vi "HEWH Decision Logic Cutout Cutin.vi"(6 "Cut Out Timer (Over)":bool, 8 "Error In":errorcluster, 9 "Bottom":bool, 10 "Cut In Timer (Over)":bool, 11 "Top":bool) -> (0 "Error Out":errorcluster, 3 "Output":bool)   [LabVIEW 2023]
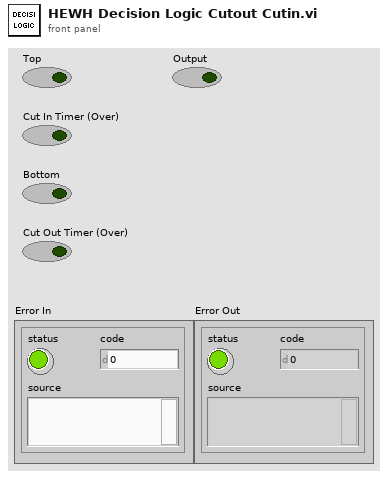
[diagram p1: front panel]
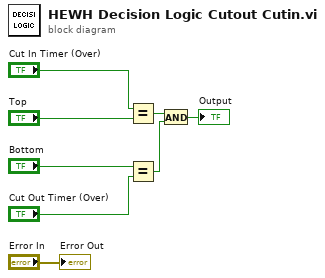
[diagram p0: block diagram]
diagram:
  n1 = Equal?(x="Cut In Timer (Over)", y="Top") -> (x = y?=w3:bool)
  n2 = Equal?(x="Bottom", y="Cut Out Timer (Over)") -> (x = y?=w2:bool)
  n3 = And(x=w3, y=w2) -> (x .and. y?=→"Output":bool)
  "Error Out" <- "Error In"
